vi "test-quintic-spline-01.vi"() -> (3 "Test Passed":bool)   [LabVIEW 2019]
uses:
  <vilib>/Rock Robotics/WPI/ThirdParty/JAS_Junk/TrajLib/POSEwCURVATURE.ctl
  <vilib>/Rock Robotics/WPI/ThirdParty/JAS_Junk/TrajLib/POSE2D.ctl
  <vilib>/Rock Robotics/WPI/ThirdParty/JAS_Junk/TrajLib/TRANSLATION2D.ctl
  <vilib>/Rock Robotics/WPI/ThirdParty/JAS_Junk/TrajLib/ROTATION2D.ctl
  <vilib>/Rock Robotics/WPI/ThirdParty/JAS_Junk/TrajLib/Rotation_CreateAngle.vi
  <vilib>/Rock Robotics/WPI/ThirdParty/JAS_Junk/TrajLib/Translation_Create.vi
  <vilib>/Rock Robotics/WPI/ThirdParty/JAS_Junk/TrajLib/Util_CalcDist.vi
  <vilib>/Rock Robotics/WPI/ThirdParty/JAS_Junk/TrajLib/Trajectory_Library.lvlib
panel:
  out "XY Graph":cluster{dbl[], dbl[]}(graph)
  out "Numb\nWaypoints":i32
  out "All Interior \nwayPoints\nFound (True)":bool
  out "end rot = 0":dbl
  out "end y = 0":dbl
  out "end x = 0":dbl
  out "start rot = 0":dbl
  out "start y = 0":dbl
  out "start x = 0":dbl
  out "max dtheta < 0.0872":dbl
  out "max dy < 0.00127":dbl
  out "max dx  < 0.127":dbl
  out "Overall Error":errorcluster
  out "Elements":i32
  out "Create Spline Error":errorcluster
  out "SplinePoses\nWCurve":T1[](array[typedef]) {"POSE"."ROTATION"."SIN" format="%13.4f"; "POSE"."ROTATION"."COS" format="%13.4f"; "POSE"."ROTATION"."VALUE" format="%13.4f"; "POSE"."TRANSLATION"."Y" format="%14.3f"; "POSE"."TRANSLATION"."X" format="%14.3f"}
  out "Elapsed Time":dbl
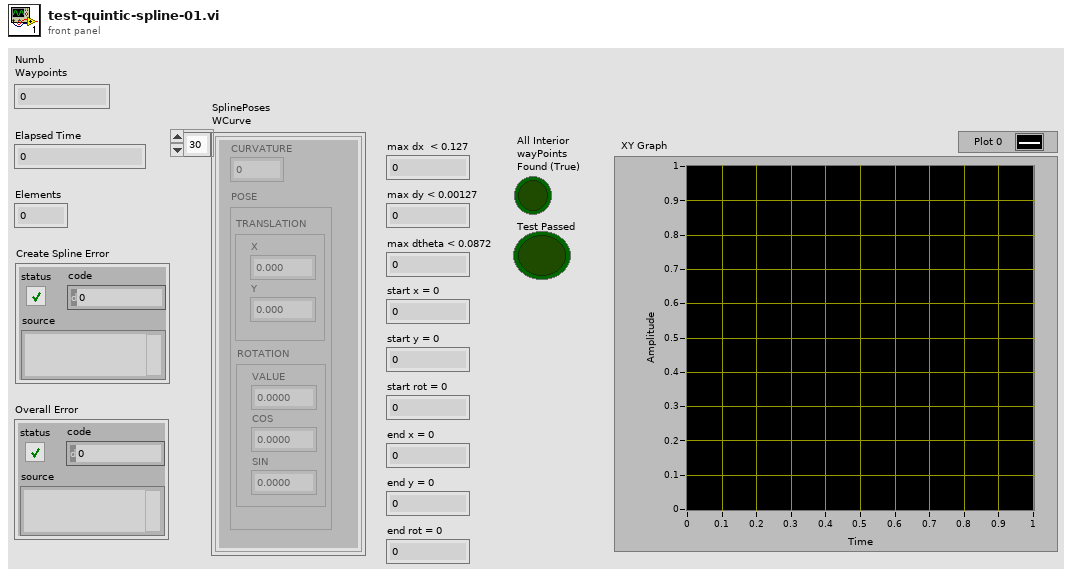
[diagram p1: front panel]
types:
  T1 = typedef "Trajectory_Library.lvlib/POSEwCURVATURE.ctl" = cluster{"CURVATURE":dbl, "POSE":T2}
  T2 = typedef "Trajectory_Library.lvlib/POSE2D.ctl" = cluster{"TRANSLATION":T3, "ROTATION":T4}
  T3 = typedef "Trajectory_Library.lvlib/TRANSLATION2D.ctl" = cluster{"X":dbl, "Y":dbl}
  T4 = typedef "Trajectory_Library.lvlib/ROTATION2D.ctl" = cluster{"VALUE":dbl, "COS":dbl, "SIN":dbl}
  T5 = typedef "Trajectory_Library.lvlib/SPLINE.ctl" = cluster{"Degree":i32, "Coefficients":T6}
  T6 = typedef "NI_Matrix.lvlib/RealMatrix.ctl" = dbl[][]
  T7 = typedef "Trajectory_Library.lvlib/TWIST2D.ctl" = cluster{"dX":dbl, "dY":dbl, "dTHETA":dbl}
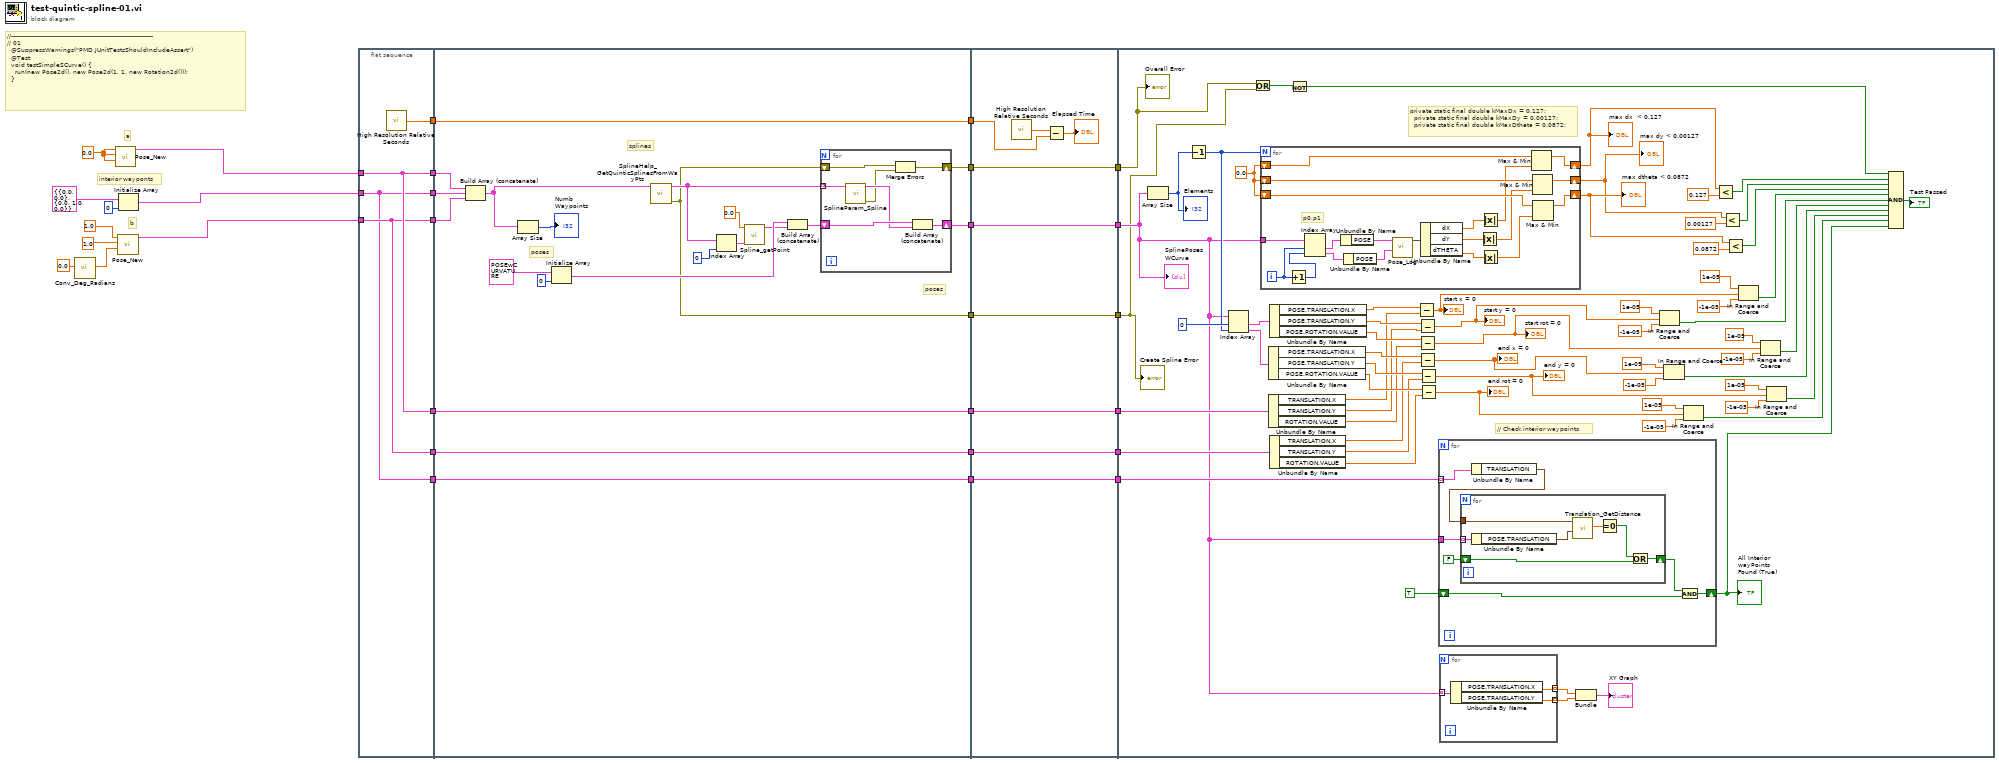
[diagram p0: block diagram]
diagram:
  w10 = 0.0 ("X")
  # "interior wayponts"
  # "b"
  # "a"
  # "//-----------------------------------------------------------------------\n// 01\n  @SuppressWarnings(\"PMD.JUnitTestsShouldIncludeAssert\")\n  @Test\n  void testSimpleSCurve() {\n    run(new Pose2d(), new Pose2d(1, 1, new Rotation2d()));\n  }"
  n1 = call <vilib>:"Conv_Deg_Radians.vi"("Degress"=0.0) -> ("Radians"=w5:dbl)  [unwired: 10 in]
  n2 = call <vilib>:"Pose_New.vi"("Heading"=w10, "Y"=w10, "X"=w10) -> ("out POSe"=w3:T2)  [unwired: 8 in]
  n3 = call <vilib>:"Pose_New.vi"("Heading"=w5, "Y"=1.0, "X"=1.0) -> ("out POSe"=w1:T2)  [unwired: 8 in]
  n4 = Initialize Array(T2 {"TRANSLATION"={"X"=0.0, "Y"=0.0}, "ROTATION"={"VALUE"=0.0, "COS"=1.0, "SIN"=0.0}} ("POSE"), 0 ("dimension size")) -> (w2:T2[])
  n5 = flat-sequence {
    tunnel: w3 -> [w33]
    tunnel: [w33] -> w30
    tunnel: w1 -> [w32]
    tunnel: [w32] -> w29
    tunnel: [w34] -> w28
    tunnel: [w33] -> w20
    tunnel: [w32] -> w17
    tunnel: [w31] -> w12
    tunnel: w2 -> [w31]
    tunnel: [w31] -> w11
    tunnel: w30 -> [w39]
    tunnel: w29 -> [w38]
    tunnel: [w55] -> w27
    tunnel: w28 -> [w55]
    tunnel: [w45] -> w26
    tunnel: [w44] -> w24
    tunnel: [w43] -> w22
    tunnel: w20 -> [w42]
    tunnel: [w42] -> w19
    tunnel: w17 -> [w41]
    tunnel: [w41] -> w16
    tunnel: [w40] -> w13
    tunnel: w12 -> [w40]
    tunnel: w11 -> [w36]
    tunnel: w27 -> [w71]
    tunnel: w26 -> [w70]
    tunnel: [w70] -> w25
    tunnel: w24 -> [w69]
    tunnel: [w69] -> w23
    tunnel: w22 -> [w68]
    tunnel: [w68] -> w21
    tunnel: w19 -> [w65]
    tunnel: [w65] -> w18
    tunnel: w16 -> [w64]
    tunnel: [w64] -> w15
    tunnel: [w63] -> w14
    tunnel: w13 -> [w63]
    tunnel: w25 -> [w112]
    tunnel: w23 -> [w99]
    tunnel: w21 -> [w98]
    tunnel: w18 -> [w134]
    tunnel: w15 -> [w133]
    tunnel: w14 -> [w116]
    frame #0 {
      n6 = call <vilib>:"High Resolution Relative Seconds.vi"() -> ("relative seconds"=w34:dbl)
    }
    frame #1 {
      # "poses"
      # "poses"
      # "splines"
      n7 = Build Array (concatenate)(w39, w36, w38) -> (w35:T2[])
      n8 = Array Size(array=w35) -> (size(s)=→"Numb\nWaypoints":i32)
      n9 = Initialize Array(T1 {"CURVATURE"=0.0, "POSE"={"TRANSLATION"={"X"=0.0, "Y"=0.0}, "ROTATION"={"VALUE"=0.0, "COS"=1.0, "SIN"=0.0}}} ("POSEwCURVATURE"), 0 ("dimension size")) -> (w49:T1[])
      n10 = call <vilib>:"SplineHelp_GetQuinticSplinesFromWayPts.vi"("WayPoints"=w35) -> ("out Error"=w44:errorcluster, "Splines"=w46:T5[])  [unwired: 9 in]
      n11 = Index Array(array=w46, index=0) -> (element=w51:T5)
      n12 = call <vilib>:"Spline_getPoint.vi"("inputSPLINE"=w51, "Time"=0.0) -> ("POSEwCURVATURE"=w48:T1)  [unwired: 9 in]
      n13 = Build Array (concatenate)(w49, w48) -> (w47:T1[])
      n14 = for {
        shift-right: [w59] -> w45
        shift-left: w47 -> [w61]
        tunnel: w46 -> [w62] mode=indexing
        shift-right: [w57] -> w43
        shift-left: w44 -> [w58]
        n15 = call <vilib>:"SplineParam_Spline.vi"("inputSPLINE"=w62) -> ("error out"=w56:errorcluster, "outputPOSEwCURVATURE"=w60:T1[])  [unwired: 9 in]
        n16 = Merge Errors(w58, w56) -> (w57:errorcluster)
        n17 = Build Array (concatenate)(w61, w60) -> (w59:T1[])
      }
    }
    frame #2 {
      n18 = call <vilib>:"High Resolution Relative Seconds.vi"() -> ("relative seconds"=w66:dbl)
      n19 = Subtract(x=w66, y=w71) -> (x-y=→"Elapsed Time":dbl)
    }
    frame #3 {
      w135 = 0.0
      # "// Check interior waypoints"
      # "private static final double kMaxDx = 0.127;\n  private static final double kMaxDy = 0.00127;\n  private static final double kMaxDtheta = 0.0872;"
      n20 = Array Size(array=w112) -> (size(s)=w136:i32)
      "Elements" <- w136
      n21 = Decrement(x=w136) -> (x-1=w131:i32)
      n22 = Index Array(array=w112, index #1=0 ("index"), index #2=w131) -> (element #1=w130:T1, element #2=w129:T1)
      n23 = Or(x=w98, y=w99) -> (x .or. y?=w100:bool)
      n24 = for {
        N: w131 -> [_]
        tunnel: w112 -> [w171]
        shift-right: [w162] -> w104
        shift-left: w135 -> [w159]
        shift-right: [w160] -> w106
        shift-left: w135 -> [w157]
        shift-right: [w161] -> w105
        shift-left: w135 -> [w158]
        i -> [w173]
        # "p0,p1"
        n25 = Increment(x=w173) -> (x+1=w172:i32)
        n26 = Index Array(array=w171, index #1=w173, index #2=w172) -> (element #1=w170:T1, element #2=w169:T1)
        n27 = Unbundle By Name(w170) -> ("POSE"=w168:T2)
        n28 = Unbundle By Name(w169) -> ("POSE"=w167:T2)
        n29 = call <vilib>:"Pose_Log.vi"("end POSE"=w167, "in POSE"=w168) -> ("out TWIST"=w166:T7)  [unwired: 9 in]
        n30 = Unbundle By Name(w166) -> ("dX"=w163:dbl, "dY"=w164:dbl, "dTHETA"=w165:dbl)
        n31 = Absolute Value(x=w164) -> (abs(x)=w155:dbl)
        n32 = Absolute Value(x=w163) -> (abs(x)=w156:dbl)
        n33 = Absolute Value(x=w165) -> (abs(x)=w154:dbl)
        n34 = Max & Min(x=w159, y=w156) -> (max(x,y)=w162:dbl)  [unwired: 1 out]
        n35 = Max & Min(x=w158, y=w155) -> (max(x,y)=w161:dbl)  [unwired: 1 out]
        n36 = Max & Min(x=w157, y=w154) -> (max(x,y)=w160:dbl)  [unwired: 1 out]
      }
      "max dx  < 0.127" <- w104
      "max dy < 0.00127" <- w105
      "max dtheta < 0.0872" <- w106
      n37 = Unbundle By Name(w129) -> ("POSE.TRANSLATION.X"=w125:dbl, "POSE.TRANSLATION.Y"=w124:dbl, "POSE.ROTATION.VALUE"=w123:dbl)
      n38 = Unbundle By Name(w134) -> ("TRANSLATION.X"=w122:dbl, "TRANSLATION.Y"=w121:dbl, "ROTATION.VALUE"=w120:dbl)
      n39 = Unbundle By Name(w130) -> ("POSE.TRANSLATION.X"=w128:dbl, "POSE.TRANSLATION.Y"=w127:dbl, "POSE.ROTATION.VALUE"=w126:dbl)
      n40 = Unbundle By Name(w133) -> ("TRANSLATION.X"=w119:dbl, "TRANSLATION.Y"=w118:dbl, "ROTATION.VALUE"=w117:dbl)
      n41 = Not(x=w100) -> (.not. x?=w97:bool)
      n42 = Subtract(x=w128, y=w122) -> (x-y=w93:dbl)
      "start x = 0" <- w93
      n43 = Subtract(x=w127, y=w121) -> (x-y=w72:dbl)
      "start y = 0" <- w72
      n44 = Subtract(x=w126, y=w120) -> (x-y=w76:dbl)
      "start rot = 0" <- w76
      n45 = Subtract(x=w125, y=w119) -> (x-y=w77:dbl)
      "end x = 0" <- w77
      n46 = Subtract(x=w124, y=w118) -> (x-y=w84:dbl)
      "end y = 0" <- w84
      n47 = Subtract(x=w123, y=w117) -> (x-y=w88:dbl)
      "end rot = 0" <- w88
      n48 = for {
        tunnel: w116 -> [w141] mode=indexing
        tunnel: w112 -> [w146]
        shift-right: [w145] -> w96
        shift-left: TRUE -> [w144]
        n49 = Unbundle By Name(w141) -> ("TRANSLATION"=w140:T3)
        n50 = for {
          tunnel: w146 -> [w150] mode=indexing
          shift-right: [w153] -> w142
          shift-left: FALSE -> [w152]
          tunnel: w140 -> [w151]
          n51 = Unbundle By Name(w150) -> ("POSE.TRANSLATION"=w149:T3)
          n52 = call <vilib>:"Translation_GetDistance.vi"("other Translation"=w149, "In Translation"=w151) -> ("Distance"=w148:dbl)  [unwired: 9 in]
          n53 = Equal To 0?(x=w148) -> (x = 0?=w147:bool)
          n54 = Or(x=w147, y=w152) -> (x .or. y?=w153:bool)
        }
        n55 = And(x=w142, y=w144) -> (x .and. y?=w145:bool)
      }
      "All Interior \nwayPoints\nFound (True)" <- w96
      n56 = for {
        tunnel: [w139] -> w114 mode=indexing
        tunnel: [w138] -> w113 mode=indexing
        tunnel: w112 -> [w137] mode=indexing
        n57 = Unbundle By Name(w137) -> ("POSE.TRANSLATION.X"=w139:dbl, "POSE.TRANSLATION.Y"=w138:dbl)
      }
      n58 = Bundle(w114, w113) -> (→"XY Graph":cluster{dbl[], dbl[]})  [unwired: 1 in]
      n59 = In Range and Coerce(upper limit=1e-05, x=w72, lower limit=-1e-05) -> (In Range?=w73:bool)  [unwired: 1 out]
      n60 = In Range and Coerce(upper limit=1e-05, x=w77, lower limit=-1e-05) -> (In Range?=w79:bool)  [unwired: 1 out]
      n61 = In Range and Coerce(upper limit=1e-05, x=w88, lower limit=-1e-05) -> (In Range?=w89:bool)  [unwired: 1 out]
      n62 = Less?(x=w104, y=0.127) -> (x < y?=w103:bool)
      n63 = Less?(x=w105, y=0.00127) -> (x < y?=w102:bool)
      n64 = Less?(x=w106, y=0.0872) -> (x < y?=w101:bool)
      n65 = In Range and Coerce(upper limit=1e-05, x=w93, lower limit=-1e-05) -> (In Range?=w92:bool)  [unwired: 1 out]
      n66 = In Range and Coerce(upper limit=1e-05, x=w76, lower limit=-1e-05) -> (In Range?=w78:bool)  [unwired: 1 out]
      n67 = In Range and Coerce(upper limit=1e-05, x=w84, lower limit=-1e-05) -> (In Range?=w85:bool)  [unwired: 1 out]
      n68 = Compound Arithmetic op=AND(w97, w103, w102, w101, w92, w73, w78, w79, w85, w89, w96) -> (→"Test Passed":bool)
      "SplinePoses\nWCurve" <- w112
      "Create Spline Error" <- w99
      "Overall Error" <- w98
    }
  }
